vi "数字转字符串.vi"(1 "填充串":string, 2 "宽度":i16, 3 "数字":dbl) -> (0 "输出":string)   [LabVIEW 2016]
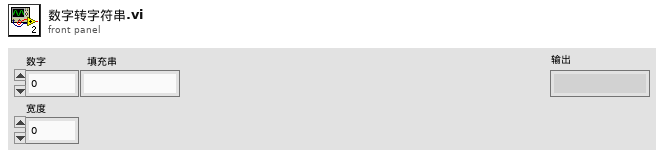
[diagram p1: front panel]
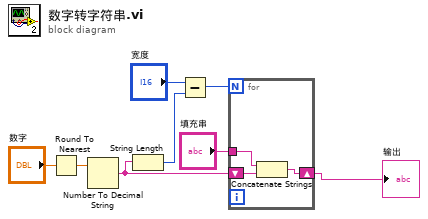
[diagram p0: block diagram]
diagram:
  n1 = Round To Nearest(number="数字") -> (nearest integer value=w8:dbl)
  n2 = Number To Decimal String(number=w8) -> (decimal integer string=w2:string)  [unwired: 1 in]
  n3 = String Length(string=w2) -> (length=w3:i32)
  n4 = Subtract(x="宽度", y=w3) -> (x-y=w6:i32)
  n5 = for {
    N: w6 -> [_]
    tunnel: "填充串" -> [w9]
    shift-right: [w11] -> w1
    shift-left: w2 -> [w10]
    n6 = Concatenate Strings(w9, w10) -> (w11:string)
  }
  "输出" <- w1
